vi "Apply Property.vi"(0 "TTLControl in":refnum<class "TTLController.lvclass">, 5 "TTL name":string, 7 "param":string, 9 "value":dbl, 11 "error in (no error)":errorcluster) -> (4 "TTLControl out":refnum<class "TTLController.lvclass">, 8 "Disabled":bool, 15 "error out":errorcluster)   [LabVIEW 2020, in "TTLController.lvclass"]
uses:
  TTLController.lvclass
  TTLController.lvclass/TTLController.ctl
  Write StopVal.vi
  Write StartVal.vi
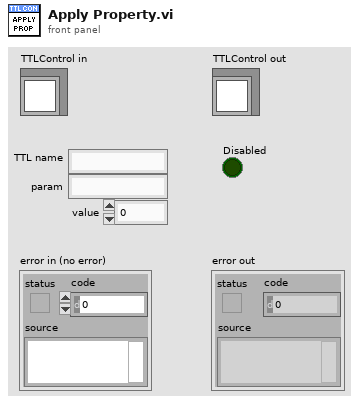
[diagram p1: front panel]
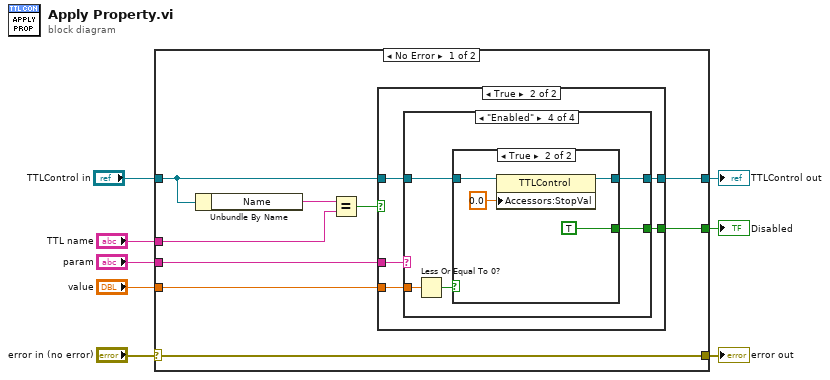
[diagram p0: block diagram]
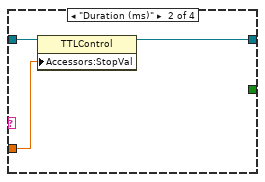
[diagram p4: hidden frame]
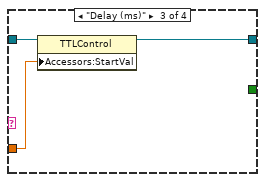
[diagram p5: hidden frame]
diagram:
  n1 = case shown="No Error" "error in (no error)" {
    selector: "error in (no error)" -> [w17 w42]
    tunnel: [w17 w42] -> w7
    tunnel: [w10 w41] -> w5
    tunnel: "TTLControl in" -> [w11 w41]
    tunnel: "TTL name" -> [w14 _]
    tunnel: "param" -> [w13 _]
    tunnel: "value" -> [w12 _]
    tunnel: [w9 _] -> w1
    frame No Error {
      n2 = Unbundle By Name(w11) -> ("Name"=w15:string)
      n3 = Equal?(x=w15, y=w14) -> (x = y?=w16:bool)
      n4 = case shown="True" w16 {
        tunnel: w11 -> [w18 w23]
        tunnel: [w18 w22] -> w10
        tunnel: w12 -> [_ w21]
        tunnel: w13 -> [_ w20]
        tunnel: [_ w19] -> w9
        frame False {
        }
        frame True {
          n5 = case shown="\"Enabled\"" w20 {
            tunnel: w23 -> [w24 w27 w30 w35]
            tunnel: [w24 w26 w29 w34] -> w22
            tunnel: w21 -> [_ w25 w28 w33]
            tunnel: [_ _ _ w31] -> w19
            frame "", Default {
            }
            frame "Duration (ms)" {
              n6 = property class="TTLControl"(reference=w27, "Accessors:StopVal"=w25) -> (reference out=w26:refnum<class "TTLController.lvclass">)  [unwired: 1 in, 1 out]
            }
            frame "Delay (ms)" {
              n7 = property class="TTLControl"(reference=w30, "Accessors:StartVal"=w28) -> (reference out=w29:refnum<class "TTLController.lvclass">)  [unwired: 1 in, 1 out]
            }
            frame "Enabled" {
              n8 = Less Or Equal To 0?(x=w33) -> (x <= 0?=w32:bool)
              n9 = case shown="True" w32 {
                tunnel: w35 -> [w36 w40]
                tunnel: [w36 w39] -> w34
                tunnel: [_ TRUE] -> w31
                frame False {
                }
                frame True {
                  n10 = property class="TTLControl"(reference=w40, "Accessors:StopVal"=0.0 ("Stop:Value")) -> (reference out=w39:refnum<class "TTLController.lvclass">)  [unwired: 1 in, 1 out]
                }
              }
            }
          }
        }
      }
    }
    frame Error {
    }
  }
  "error out" <- w7
  "TTLControl out" <- w5
  "Disabled" <- w1
